vi "Global_CMD.vi"() -> ()   [LabVIEW 2017, in "Lift.lvlib"]
uses:
  Lift.lvlib
  CLUSTER_CMD_SM_Lift_Rotate.ctl
  ENUM_SM_Rotate_Positions.ctl
panel:
  in  "CMD_SM_Lift":T1={"Enable System"=TRUE, "Rotate Position"=enum."Neutral: 0", "Manual Velocity"=0.0, "Manual Mode"=FALSE, "Manual Override"=FALSE}
  # "The Names of the Data items in the Global Variable MUST describe who the Single Writer is\nNaming Convention for Command Globals is:   \n\nCMD_SubSystem_Data Name\nExample:\nCMD_Drive_Mode\nCMD_Hopper_Fire Ball"
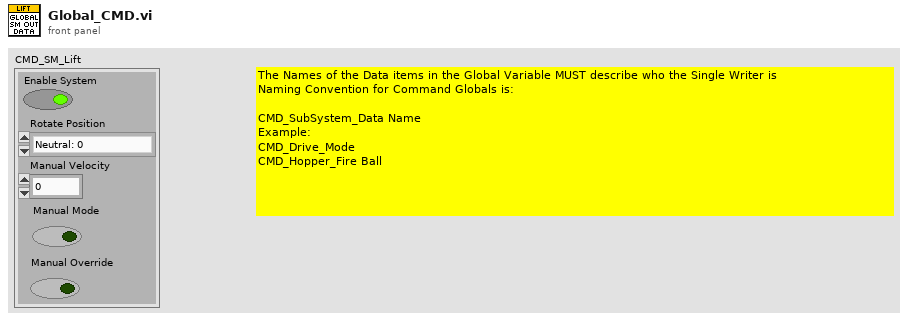
[diagram p1: front panel]
types:
  T1 = typedef "Lift.lvlib/CLUSTER_CMD_SM_Lift_Rotate.ctl" = cluster{"Enable System":bool, "Rotate Position":T2, "Manual Velocity":dbl, "Manual Mode":bool, "Manual Override":bool}
  T2 = typedef "Lift.lvlib/ENUM_SM_Rotate_Positions.ctl" = enum16{"Neutral: 0", "Pickup: 0", "Exchange: 0", "Switch: 0", "Scale: 0", "Climb: 0"}
diagram:
